vi "Practica_Medicion_Remota.vi"() -> ()   [LabVIEW 2020]
uses:
  <vilib>/httpClient/LabVIEWHTTPClient.lvlib
panel:
  out "Led Rele":bool
  out "Hora":string
  out "Data":string
  out "Feedback [mA]":dbl
  out "error out":errorcluster
  out "body":string
  out "headers":string
  in  "stop":bool
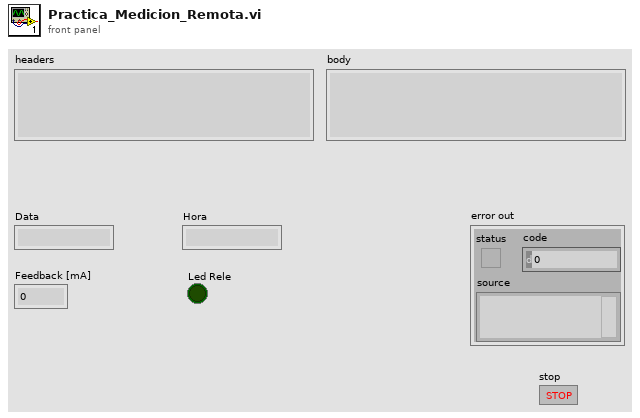
[diagram p1: front panel]
types:
  T1 = cluster{"Accionamiento":dbl, "Data":string, "Hora":string, "Rele":bool}
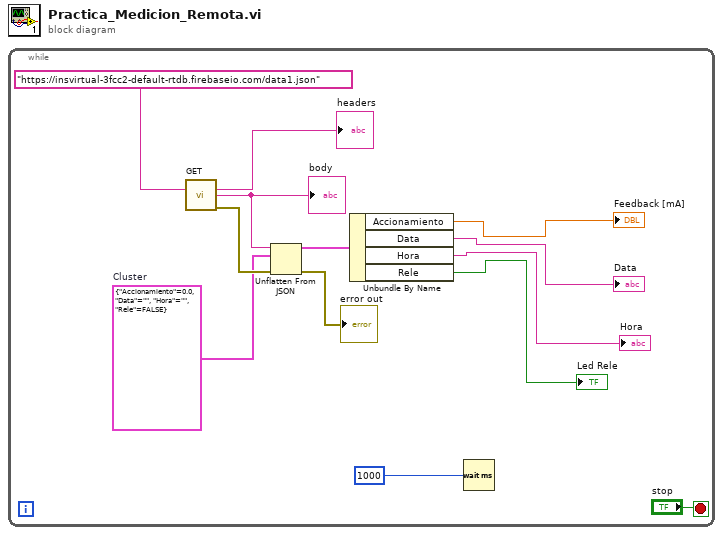
[diagram p0: block diagram]
diagram:
  n1 = while {
    stop <- "stop" stop-if-true
    w6 = T1 {"Accionamiento"=0.0, "Data"="", "Hora"="", "Rele"=FALSE}  # Cluster
    n2 = call <vilib>:"GET.vi"("url"="https://insvirtual-3fcc2-default-rtdb.firebaseio.com/data1.json") -> ("headers"=→"headers":string, "body"=w7:string, "error out"=w8:errorcluster)  [unwired: 11 in, 1 out]
    "body" <- w7
    n3 = Unflatten From JSON(JSON string=w7, type and defaults=w6, error in (no error)=w8) -> (value=w5:T1, error out=→"error out":errorcluster)  [unwired: 4 in]
    n4 = Unbundle By Name(w5) -> ("Accionamiento"=→"Feedback [mA]":dbl, "Data"=→"Data":string, "Hora"=→"Hora":string, "Rele"=→"Led Rele":bool)
    n5 = Wait (ms)(milliseconds to wait=u32 1000) -> ()  [unwired: 1 out]
  }
